vi "ZeroMQ_module.vi"   [LabVIEW 2020]
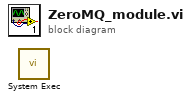
[diagram p0: block diagram]
diagram:
  n1 = call <vilib>:"System Exec.vi"() -> ()  [unwired: 8 in, 4 out]
